vi "Get Current Log File Instance Data.vi"(8 "error in (no error)":errorcluster, 11 "Segmented Log in":refnum<class "Segmented Log.lvclass">) -> (0 "error out":errorcluster, 2 "File Instance Data":T1, 3 "Segmented Log out":refnum<class "Segmented Log.lvclass">)   [LabVIEW 2015, in "Waveform Data Logger Engine.lvlib" / "Segmented Log.lvclass"]
uses:
  Segmented Log.lvclass
  File Instance Data.ctl
  Segmented Log.lvclass/Segmented Log.ctl
  Log Files/Log File/Log File.lvclass/Log File.ctl
  Log Files/Log File/Log File.lvclass
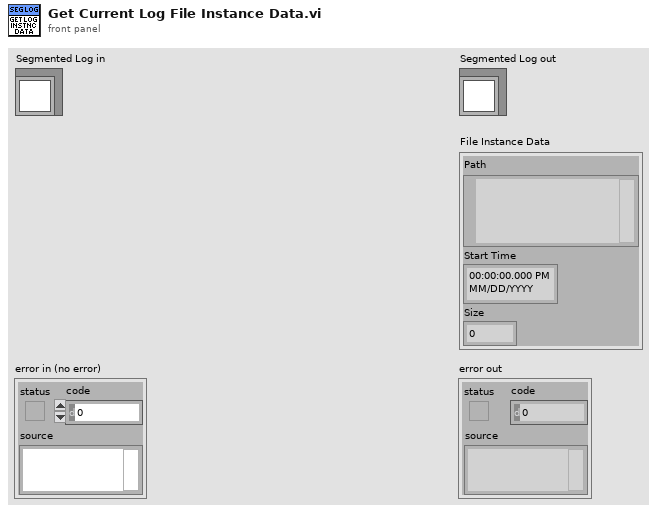
[diagram p1: front panel]
types:
  T1 = typedef "Waveform Data Logger Engine.lvlib/Segmented Log.lvclass/File Instance Data.ctl" = cluster{"Path":path, "Start Time":timestamp, "Size":i64}
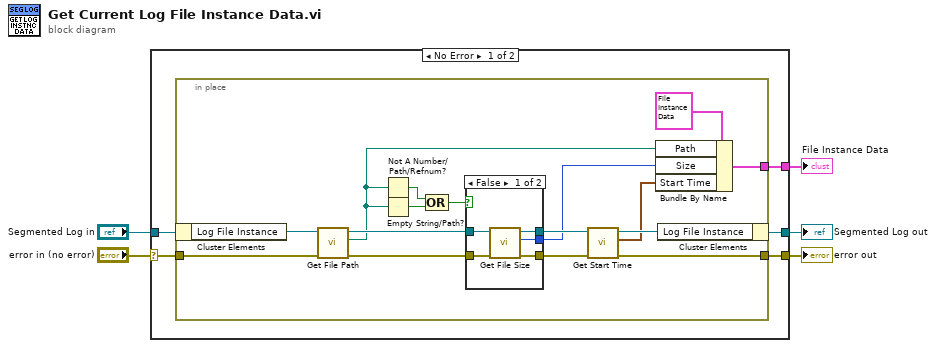
[diagram p0: block diagram]
diagram:
  n1 = case shown="No Error" "error in (no error)" {
    selector: "error in (no error)" -> [w9 w35]
    tunnel: [w7 w35] -> w4
    tunnel: [w8 w34] -> w2
    tunnel: "Segmented Log in" -> [w10 w34]
    tunnel: [w6 _] -> w1
    frame No Error {
      n2 = in-place {
        in-place-border: w9 -> [w24]
        in-place-border: [w15] -> w7
        in-place-border: [w22] -> w6
        n3 = in-place-cluster #1(w10) -> ("Log File Instance"=w25:refnum<class "Log File.lvclass">)
        n4 = call "Get File Path.vi"("error in (no error)"=w24, "Log File in"=w25) -> ("error out"=w12:errorcluster, "File Path"=w19:path, "Log File out"=w26:refnum<class "Log File.lvclass">)  [unwired: 7 in]
        n5 = Not A Number/Path/Refnum?(number/path/refnum=w19) -> (NaN/Path/Refnum?=w21:bool)
        n6 = Empty String/Path?(string/path=w19) -> (empty?=w20:bool)
        n7 = Compound Arithmetic op=OR(w21, w20) -> (w18:bool)
        n8 = case shown="False" w18 {
          tunnel: w26 -> [w31 w33]
          tunnel: w12 -> [w30 w32]
          tunnel: [w29 w33] -> w14
          tunnel: [w28 w32] -> w13
          tunnel: [w27 _] -> w11
          frame False {
            n9 = call "Get File Size.vi"("error in (no error)"=w30, "Log File in"=w31) -> ("error out"=w28:errorcluster, "size (in bytes)"=w27:i64, "Log File out"=w29:refnum<class "Log File.lvclass">)  [unwired: 7 in]
          }
          frame True {
          }
        }
        n10 = call "Get Start Time.vi"("error in (no error)"=w13, "Log File in"=w14) -> ("error out"=w15:errorcluster, "Start Time"=w16:timestamp, "Log File out"=w17:refnum<class "Log File.lvclass">)  [unwired: 7 in]
        n11 = Bundle By Name(cluster=T1 {"Path"=path "", "Start Time"=timestamp(0 s since 1904-01-01), "Size"=0} ("File Instance Data"), "Path"=w19, "Size"=w11, "Start Time"=w16) -> (w22:T1)
        n12 = in-place-cluster #1("Log File Instance"=w17) -> (w8:refnum<class "Segmented Log.lvclass">)
      }
    }
    frame Error {
    }
  }
  "error out" <- w4
  "Segmented Log out" <- w2
  "File Instance Data" <- w1
